vi "Configure TCP Connection.vi"(4 "Read Mode (Immediate)":T1(ring)=enum."Immediate", 5 "Connection.TCP":refnum<class "Connection.TCP.lvclass">, 6 "timeout (5000ms)":i32=5000, 8 "error in (no error)":errorcluster, 10 "remote port (80)":u16=80, 11 "address (localhost)":string="localhost") -> (0 "error out":errorcluster, 3 "Connection.TCP":refnum<class "Connection.TCP.lvclass">)   [LabVIEW 2013, in "Connection.TCP_GOSPL.lvlib" / "Connection.TCP.lvclass"]
uses:
  Connection.TCP.lvclass
  Connection.TCP.lvclass/Connection.TCP.ctl
  Connection/Connection.lvclass/Connection.ctl
  Connection/Connection.lvclass
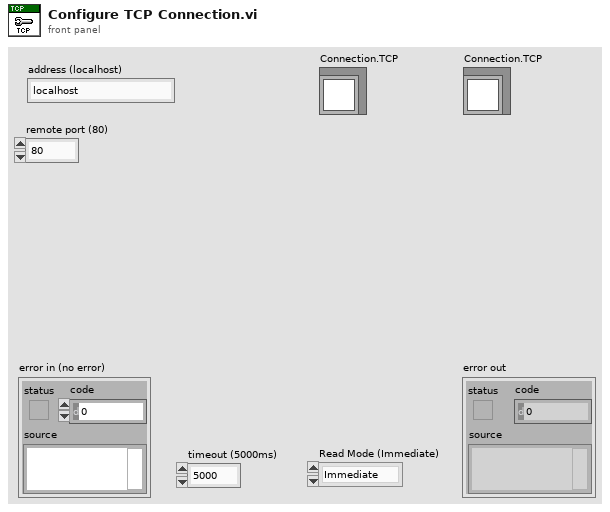
[diagram p1: front panel]
types:
  T1 = enum16{"Standard", "Buffered", "CRLF", "Immediate"}
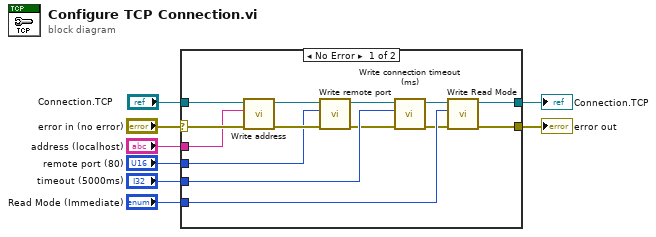
[diagram p0: block diagram]
diagram:
  n1 = case shown="No Error" "error in (no error)" {
    selector: "error in (no error)" -> [w11 w24]
    tunnel: [w17 w24] -> w7
    tunnel: [w19 w23] -> w3
    tunnel: "address (localhost)" -> [w9 _]
    tunnel: "remote port (80)" -> [w10 _]
    tunnel: "timeout (5000ms)" -> [w22 _]
    tunnel: "Read Mode (Immediate)" -> [w21 _]
    tunnel: "Connection.TCP" -> [w16 w23]
    frame No Error {
      n2 = call "Write address.vi"("error in (no error)"=w11, "address"=w9, "Connection.TCP"=w16) -> ("error out"=w12:errorcluster, "Connection.TCP"=w15:refnum<class "Connection.TCP.lvclass">)  [unwired: 7 in]
      n3 = call "Write remote port.vi"("error in (no error)"=w12, "remote port (80)"=w10, "Connection.TCP"=w15) -> ("error out"=w13:errorcluster, "Connection.TCP"=w14:refnum<class "Connection.TCP.lvclass">)  [unwired: 7 in]
      n4 = call "Write connection timeout (ms).vi"("error in (no error)"=w13, "connection timeout (ms)"=w22, "Connection in"=w14) -> ("error out"=w18:errorcluster, "Connection out"=w20:refnum<class "Connection.TCP.lvclass">)  [unwired: 7 in]
      n5 = call "Write Read Mode.vi"("error in (no error)"=w18, "Read Mode"=w21, "Connection.TCP"=w20) -> ("error out"=w17:errorcluster, "Connection.TCP"=w19:refnum<class "Connection.TCP.lvclass">)  [unwired: 7 in]
    }
    frame Error {
    }
  }
  "error out" <- w7
  "Connection.TCP" <- w3
